vi "FGV Slit.vi"(8 "error in (no error)":errorcluster, 10 "FGV Slit Data In":T1 {"Système ID" min=1 max=10 step=1; "Portnumber" items=["COM1", "COM2", "COM3", "COM4", "COM5", "COM6", "COM7", "COM8", "COM9", "COM10", "COM11", "COM12", "COM13", "COM14", "COM15", "COM16", "COM17", "COM18", "COM19", "COM20", "COM21", "COM22", "COM23", "COM24", "COM25", "COM26", "COM27", "COM28", "COM29", "COM30"]}, 11 "Action":T2) -> (0 "error out":errorcluster, 3 "FGV Slit Data Out":T1={"Portnumber"=0, "Position"=0.0, "Status"="", "Système ID"=1, "Connected axes"=[], "Velocity"=0.0, "Stage names"=[], "Device ID out"=0} {"Système ID" min=1 max=10 step=1; "Portnumber" items=["COM1", "COM2", "COM3", "COM4", "COM5", "COM6", "COM7", "COM8", "COM9", "COM10", "COM11", "COM12", "COM13", "COM14", "COM15", "COM16", "COM17", "COM18", "COM19", "COM20", "COM21", "COM22", "COM23", "COM24", "COM25", "COM26", "COM27", "COM28", "COM29", "COM30"]})   [LabVIEW 2017]
uses:
  Action Slit.ctl
  FGV Slit Data.ctl
  <userlib>/GCSLabView/Low Level/Communication.llb/Available interfaces.ctl
  <userlib>/GCSLabView/Low Level/Communication.llb/Available DLLs.ctl
  <userlib>/GCSLabView/Low Level/Communication.llb/Available DLL interfaces.ctl
  <userlib>/GCSLabView/Low Level/General command.llb/Controller names.ctl
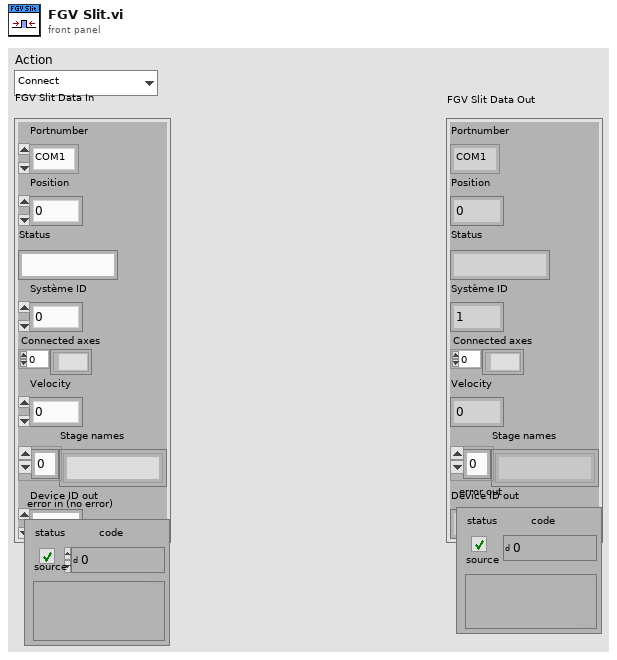
[diagram p1: front panel]
types:
  T1 = typedef "FGV Slit Data.ctl" = cluster{"Portnumber":i32, "Position":dbl, "Status":string, "Système ID":i32, "Connected axes":string[], "Velocity":dbl, "Stage names":string[], "Device ID out":i32}
  T2 = typedef "Action Slit.ctl" = enum16{"Connect", "Initialize", "Set Velocity", "Get Velocity", "Move Rel", "Move Abs", "Position", "Status", "Abort", "Disconnect"}
  T3 = typedef "Available interfaces.ctl" = u16
  T4 = cluster{"RS232 Portnumber":i32, "Timeout":i32, "RS232 Baud rate":u32, "Interface":T3, "GPIB Bus":i32, "GPIB Address":i32, "GPIB Mode":i32}
  T5 = cluster{"input XON/XOFF":bool, "input HW Handshake":bool, "input alt HW HShk":bool, "output XON/XOFF":bool, "output HW Handshake":bool, "output alt HW HShk":bool, "XOFF byte ":u8, "XON byte":u8, "parity error byte":u16}
  T6 = cluster{"data bits":u16, "stop bits":enum16{"1 bit", "1.5 bits", "2 bits"}, "parity":enum16{"no parity", "odd parity", "even parity", "mark parity", "space parity"}}
  T7 = typedef "Controller names.ctl" = enum16{"None", "Analog", "C-702", "C-843", "C-843.PM", "C-844", "C-848", "C-865", "C-866", "C-867", "C-880", "E-516", "E-517", "E-709", "E-710", "E-712", "E-725", "E-753", "E-755", "E-761", "E-816", "E-861", "F-206", "M-840", "M-850", "M-8X0", "Mercury", "Mercury_GCS"}
  T8 = typedef "Available DLLs.ctl" = u16
  T9 = typedef "Available DLL interfaces.ctl" = u16
  T10 = cluster{"DLL for Device":T8, "DLL Interface":T9, "Parameter":string}
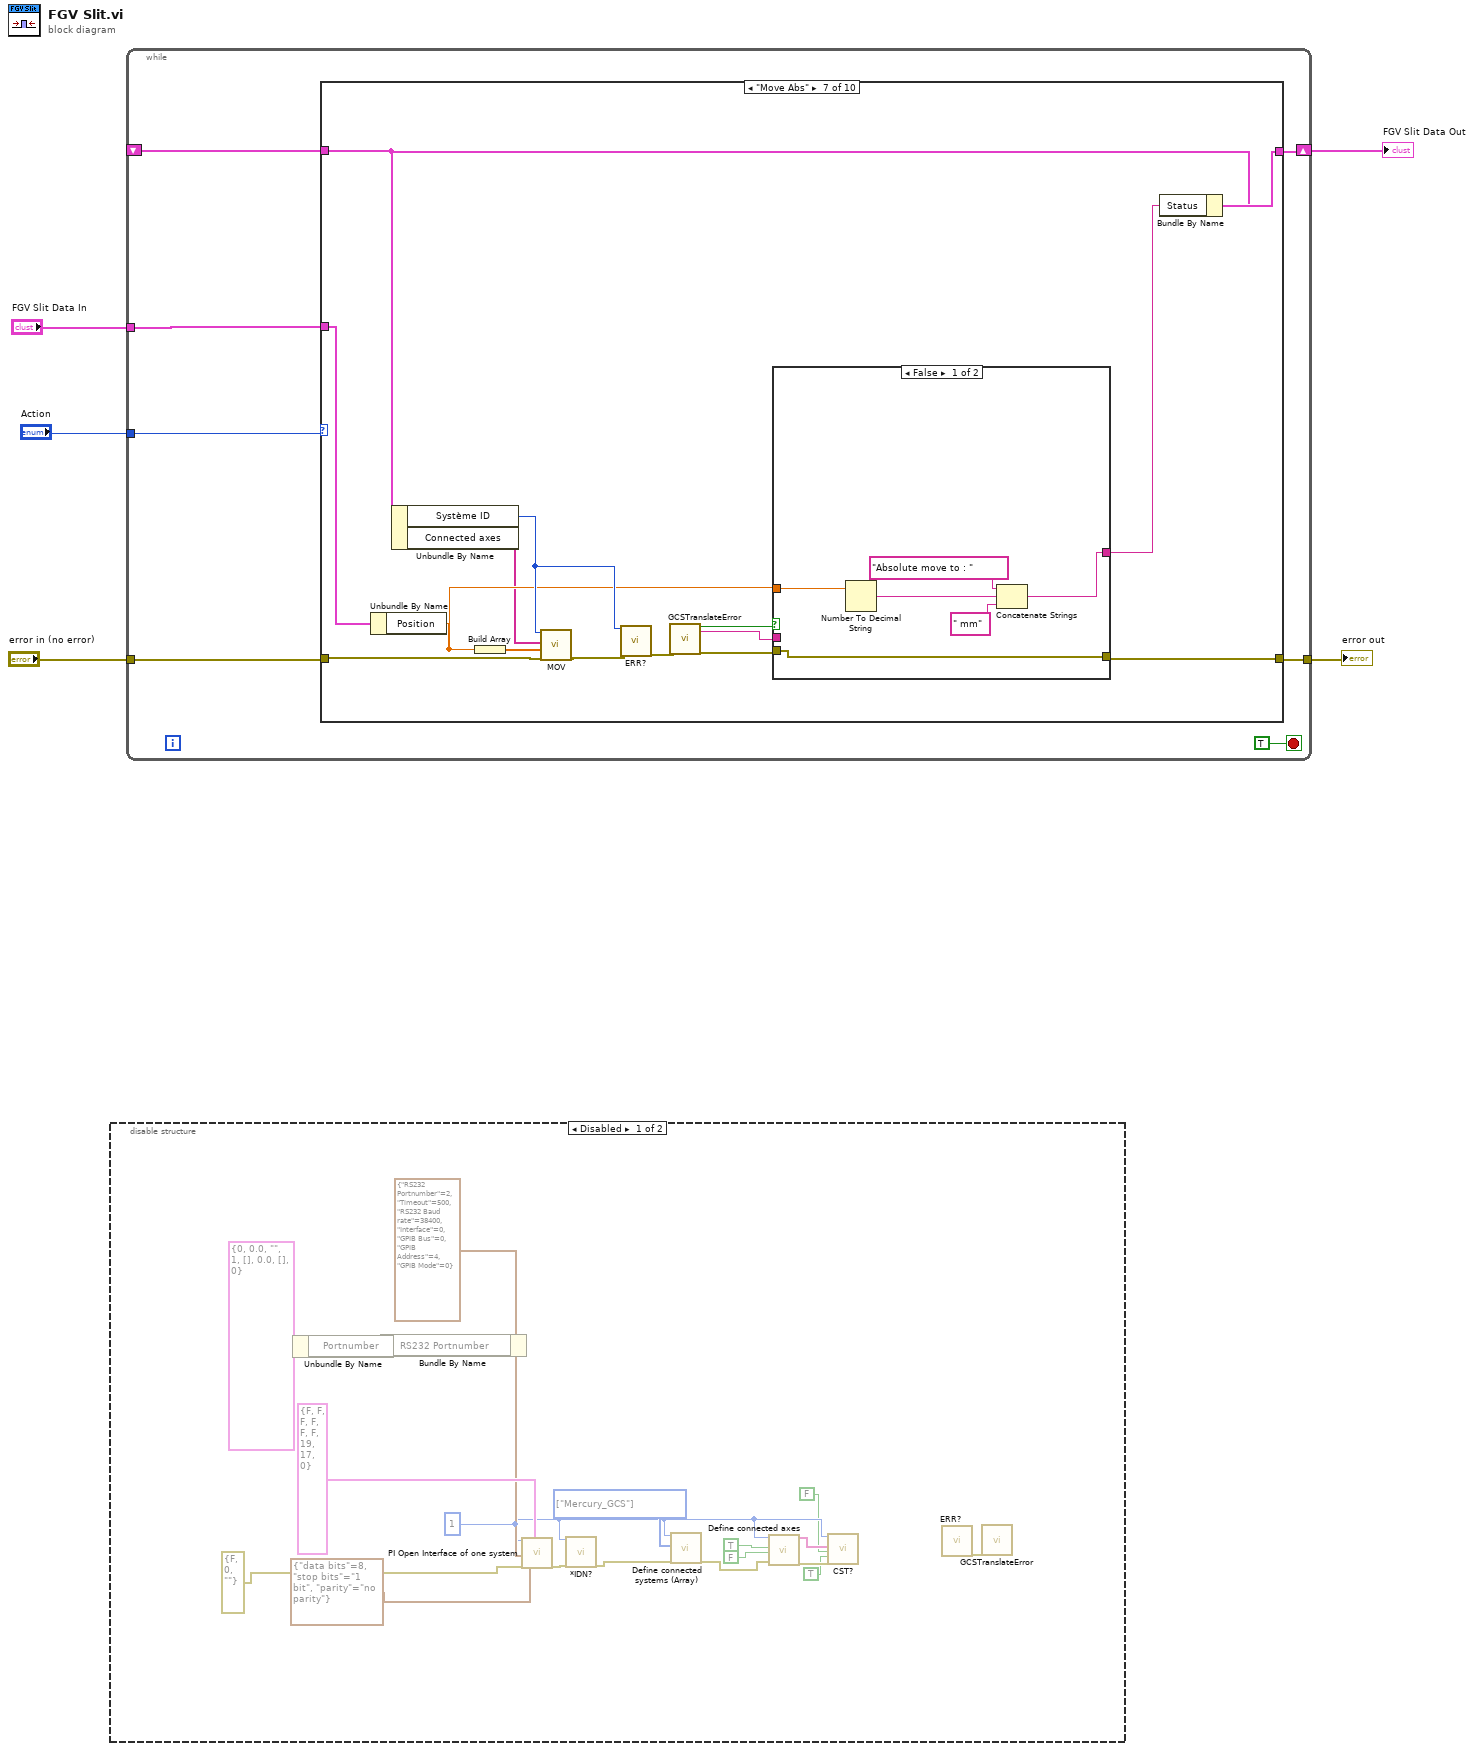
[diagram p0: block diagram]
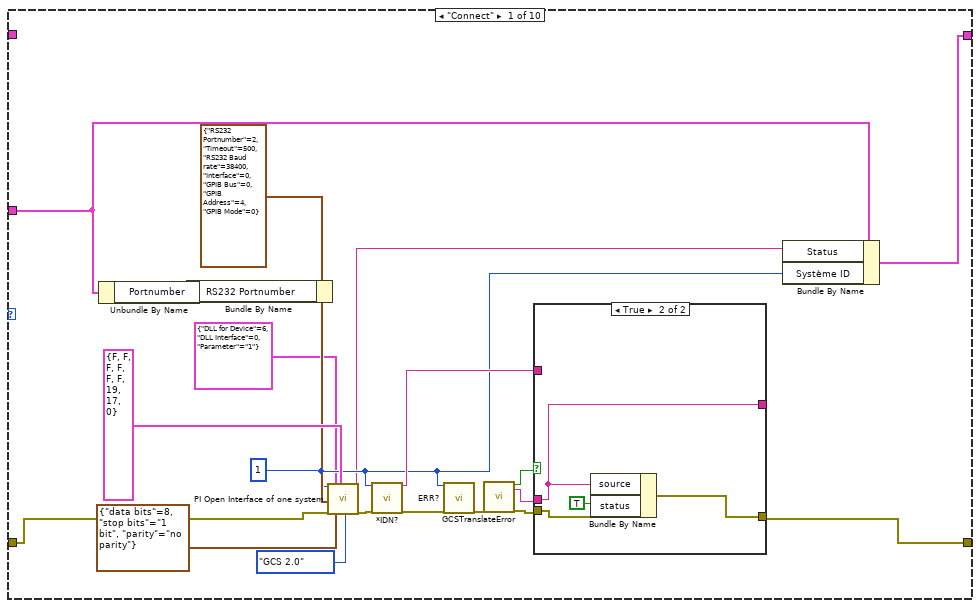
[diagram p3: hidden frame]
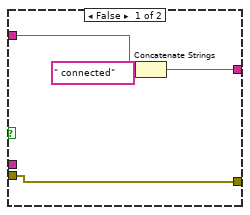
[diagram p4: hidden frame]
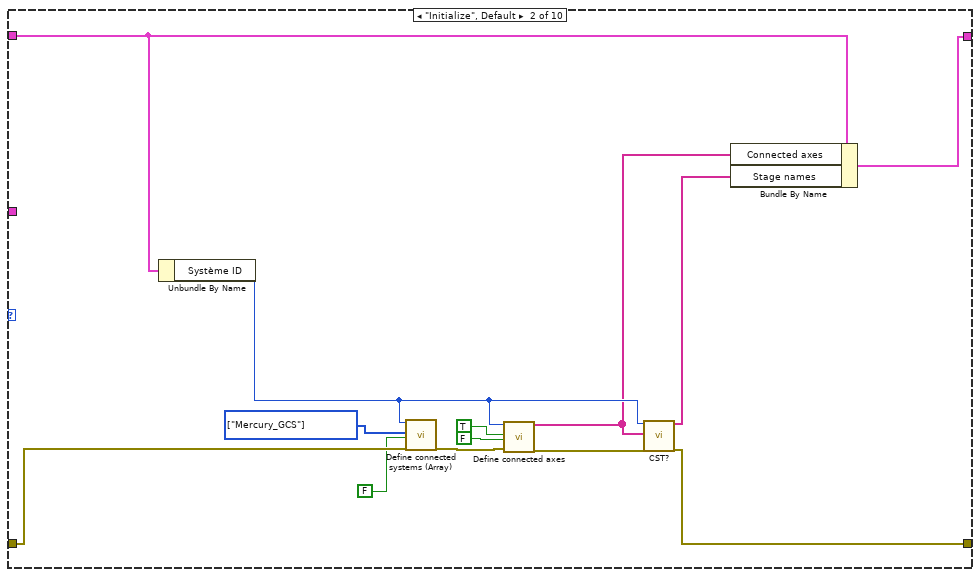
[diagram p5: hidden frame]
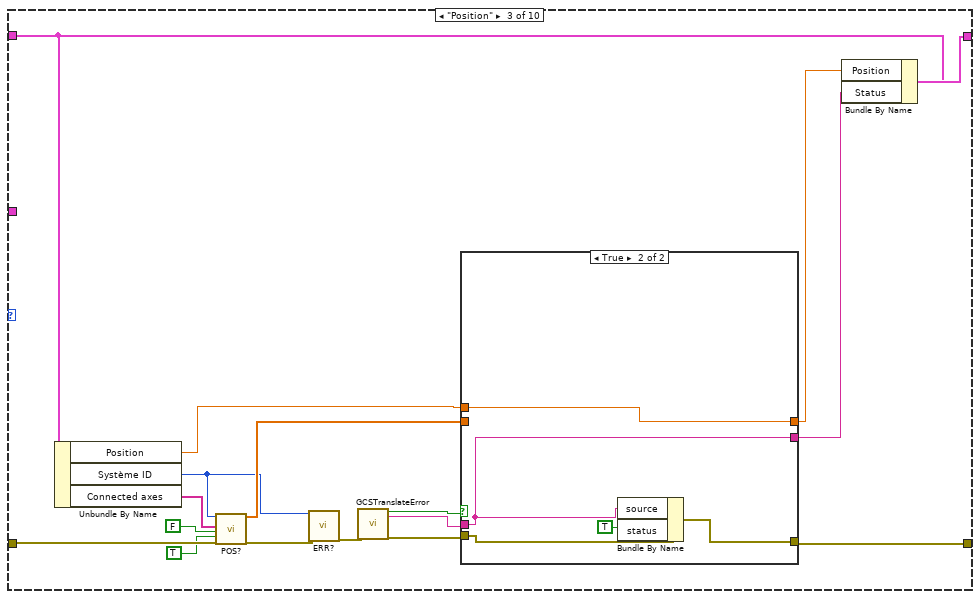
[diagram p6: hidden frame]
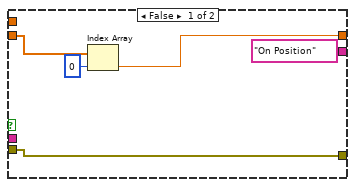
[diagram p7: hidden frame]
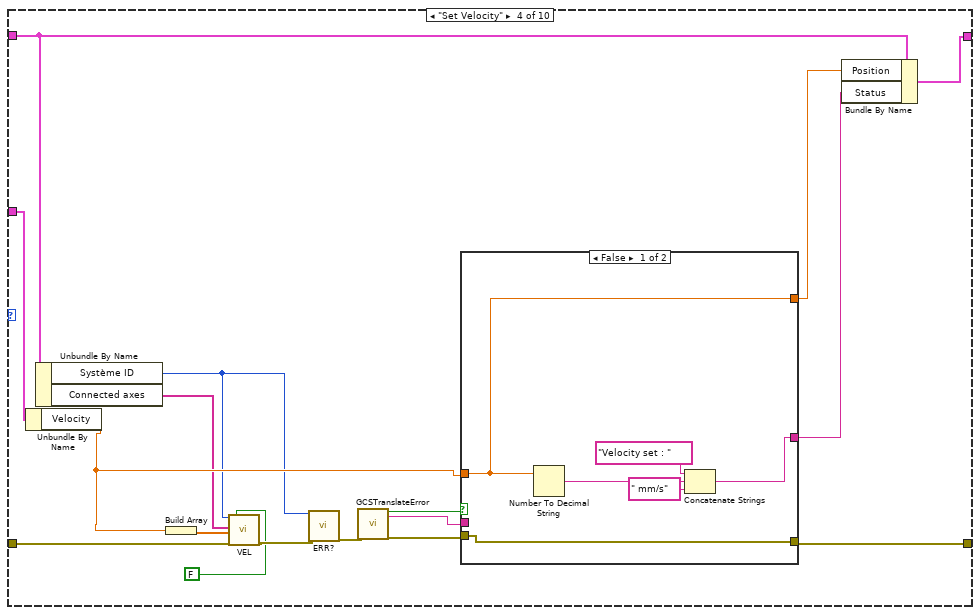
[diagram p8: hidden frame]
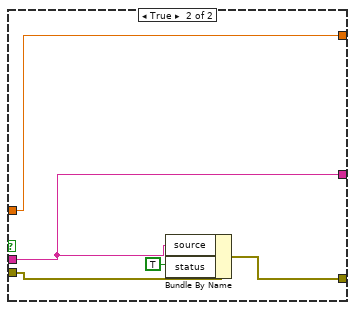
[diagram p9: hidden frame]
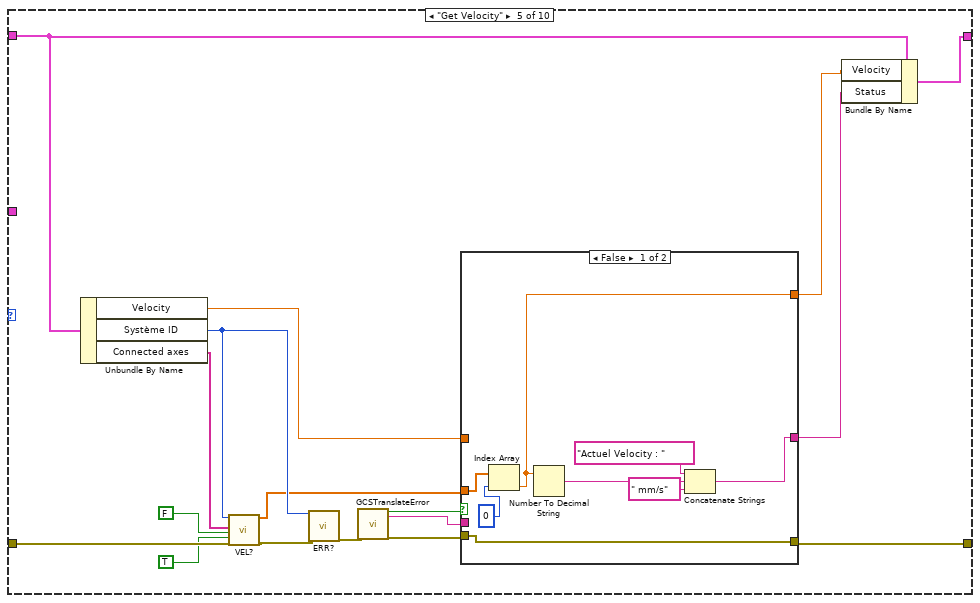
[diagram p10: hidden frame]
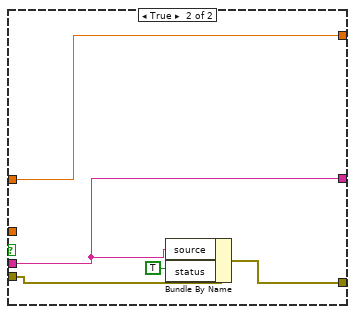
[diagram p11: hidden frame]
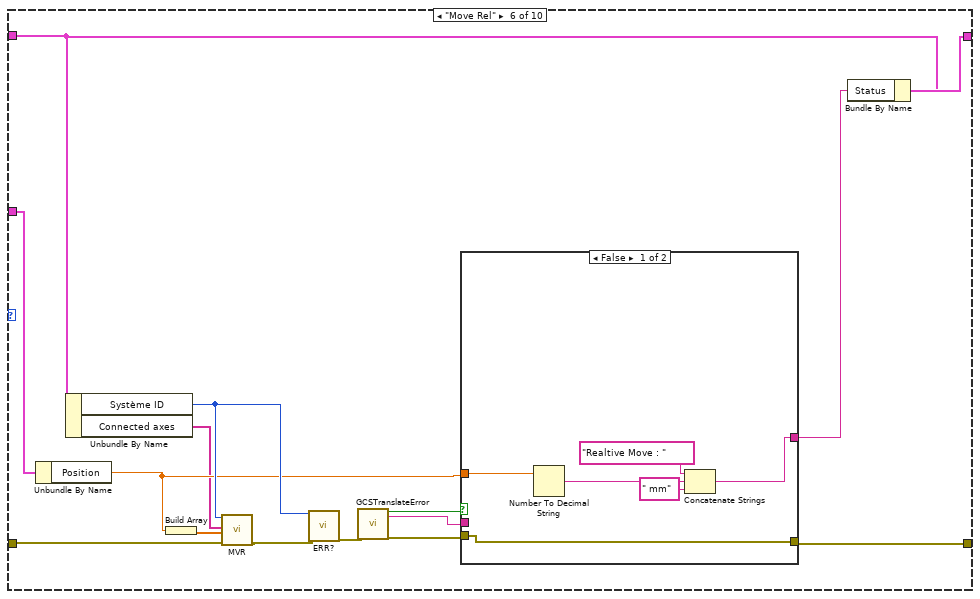
[diagram p12: hidden frame]
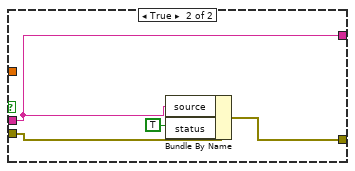
[diagram p13: hidden frame]
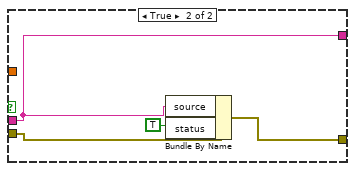
[diagram p14: hidden frame]
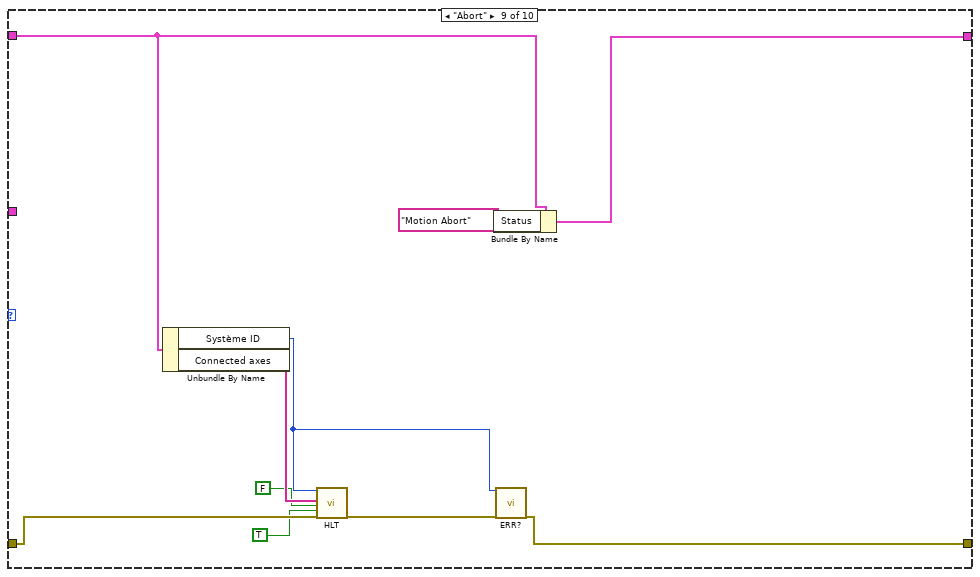
[diagram p16: hidden frame]
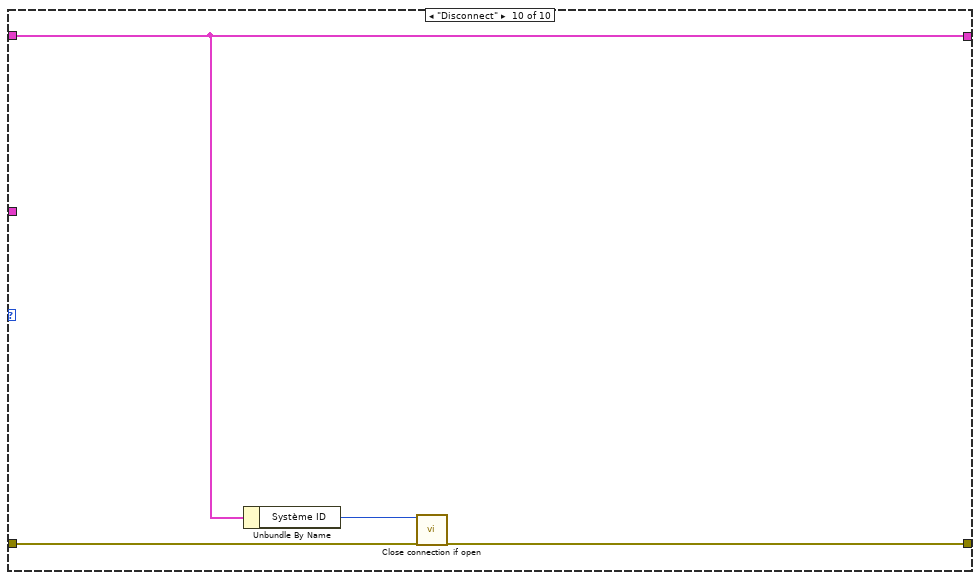
[diagram p17: hidden frame]
diagram:
  n1 = disable-structure shown="Disabled" {
    frame Disabled {
      w18 = T7[] [enum."Mercury_GCS"] items=["None", "Analog", "C-702", "C-843", "C-843.PM", "C-844", "C-848", "C-865", "C-866", "C-867", "C-880", "E-516", "E-517", "E-709", "E-710", "E-712", "E-725", "E-753", "E-755", "E-761", "E-816", "E-861", "F-206", "M-840", "M-850", "M-8X0", "Mercury", "Mercury_GCS"] ("Controller names")
      w10 = 1 ("System number")
      n2 = Unbundle By Name(T1 {"Portnumber"=0, "Position"=0.0, "Status"="", "Système ID"=1, "Connected axes"=[], "Velocity"=0.0, "Stage names"=[], "Device ID out"=0} ("input cluster")) -> ("Portnumber"=w20:i32)
      n3 = Bundle By Name(cluster=T4 {"RS232 Portnumber"=2, "Timeout"=500, "RS232 Baud rate"=38400, "Interface"=0, "GPIB Bus"=0, "GPIB Address"=4, "GPIB Mode"=0} ("Interface configuration"), "RS232 Portnumber"=w20) -> (w19:T4)
      n4 = call <userlib>:"PI Open Interface of one system.vi"("System number"=w10, "Interface configuration"=w19, "error in"=errorcluster {"status"=FALSE, "code"=0, "source"=""}, "Bit settings and parity"=T6 {"data bits"=8, "stop bits"=enum."1 bit", "parity"=enum."no parity"}, "Flow control"=T5 {"input XON/XOFF"=FALSE, "input HW Handshake"=FALSE, "input alt HW HShk"=FALSE, "output XON/XOFF"=FALSE, "output HW Handshake"=FALSE, "output alt HW HShk"=FALSE, "XOFF byte "=19, "XON byte"=17, "parity error byte"=0}) -> ("error out"=w22:errorcluster)  [unwired: 13 in, 1 out]
      n5 = call <userlib>:"*IDN?.vi"("System no."=w10, "error in"=w22) -> ("error out"=w14:errorcluster)  [unwired: 16 in, 1 out]
      n6 = call <userlib>:"Define connected systems (Array).vi"("System no."=w10, "Controller names"=w18, "error in"=w14) -> ("error out"=w11:errorcluster)  [unwired: 16 in]
      n7 = call <userlib>:"Define connected axes.vi"("System no."=w10, "Read from\ncontroller?"=TRUE ("Read from\ncontroller?"), "Invert\norder?"=FALSE ("Invert\norder?"), "error in"=w11) -> ("Conn. Axes out"=w9:string[], "error out"=w8:errorcluster)  [unwired: 14 in]
      n8 = call <userlib>:"CST?.vi"("System no."=w10, "Axes to query"=w9, "All Axes?"=FALSE, "Axis Identifier?"=TRUE, "error in"=w8) -> ()  [unwired: 13 in, 2 out]
      n9 = call <userlib>:"ERR?.vi"() -> ("error out"=w24:errorcluster)  [unwired: 18 in, 1 out]
      n10 = call <userlib>:"GCSTranslateError.vi"("error in"=w24) -> ()  [unwired: 16 in, 3 out]
    }
    frame Enabled {
    }
  }
  n11 = while {
    tunnel: "Action" -> [w30]
    tunnel: "FGV Slit Data In" -> [w29]
    shift-right: [w28] -> w3
    shift-left: _ -> [w25]
    tunnel: "error in (no error)" -> [w27]
    tunnel: [w26] -> w1
    stop <- TRUE stop-if-true
    n12 = case shown="\"Move Abs\"" w30 {
      tunnel: w29 -> [w48 _ _ w105 _ w160 w185 _ _ _]
      tunnel: [w50 w62 w85 w112 w140 w168 w193 w209 w213 w222] -> w28
      tunnel: w25 -> [_ w64 w81 w102 w130 w161 w186 w209 w215 w222]
      tunnel: w27 -> [w49 w67 w83 w108 w136 w165 w189 w208 w219 w223]
      tunnel: [w51 w66 w84 w111 w139 w167 w192 w208 w217 w220] -> w26
      frame "Connect" {
        w36 = 1 ("System number")
        n13 = Unbundle By Name(w48) -> ("Portnumber"=w38:i32)
        n14 = Bundle By Name(cluster=T4 {"RS232 Portnumber"=2, "Timeout"=500, "RS232 Baud rate"=38400, "Interface"=0, "GPIB Bus"=0, "GPIB Address"=4, "GPIB Mode"=0} ("Interface configuration"), "RS232 Portnumber"=w38) -> (w37:T4)
        n15 = call <userlib>:"PI Open Interface of one system.vi"("System number"=w36, "Interface configuration"=w37, "error in"=w49, "DLL Interface\nConfiguration"=T10 {"DLL for Device"=6, "DLL Interface"=0, "Parameter"="1"} ("DLL Interface\nConfiguration"), "Bit settings and parity"=T6 {"data bits"=8, "stop bits"=enum."1 bit", "parity"=enum."no parity"}, "Flow control"=T5 {"input XON/XOFF"=FALSE, "input HW Handshake"=FALSE, "input alt HW HShk"=FALSE, "output XON/XOFF"=FALSE, "output HW Handshake"=FALSE, "output alt HW HShk"=FALSE, "XOFF byte "=19, "XON byte"=17, "parity error byte"=0}, "Syntax"=enum16{"GCS 1.0", "GCS 2.0"}."GCS 2.0") -> ("String read"=w33:string, "error out"=w41:errorcluster)  [unwired: 11 in]
        n16 = call <userlib>:"*IDN?.vi"("System no."=w36, "error in"=w41) -> ("Identification"=w40:string, "error out"=w35:errorcluster)  [unwired: 16 in]
        n17 = call <userlib>:"ERR?.vi"("System no."=w36, "error in"=w35) -> ("error out"=w47:errorcluster)  [unwired: 16 in, 1 out]
        n18 = call <userlib>:"GCSTranslateError.vi"("error in"=w47) -> ("GCS Error?"=w46:bool, "Error Description"=w45:string, "error out"=w44:errorcluster)  [unwired: 16 in]
        n19 = case shown="True" w46 {
          tunnel: w40 -> [w55 _]
          tunnel: [w52 w58] -> w51
          tunnel: [w53 w57] -> _
          tunnel: w45 -> [_ w57]
          tunnel: w44 -> [w52 w59]
          frame False {
            n20 = Concatenate Strings(w55, " connected" ("string")) -> (w53:string)
          }
          frame True {
            n21 = Bundle By Name(cluster=w59, "source"=w57, "status"=TRUE) -> (w58:errorcluster)
          }
        }
        n22 = Bundle By Name(cluster=w48, "Status"=w33, "Système ID"=w36) -> (w50:T1)
      }
      frame "Initialize", Default {
        w72 = T7[] [enum."Mercury_GCS"] items=["None", "Analog", "C-702", "C-843", "C-843.PM", "C-844", "C-848", "C-865", "C-866", "C-867", "C-880", "E-516", "E-517", "E-709", "E-710", "E-712", "E-725", "E-753", "E-755", "E-761", "E-816", "E-861", "F-206", "M-840", "M-850", "M-8X0", "Mercury", "Mercury_GCS"] ("Controller names")
        n23 = Unbundle By Name(w64) -> ("Système ID"=w65:i32)
        n24 = call <userlib>:"Define connected systems (Array).vi"("System no."=w65, "Controller names"=w72, "Change only one system?"=FALSE, "error in"=w67) -> ("error out"=w69:errorcluster)  [unwired: 15 in]
        n25 = call <userlib>:"Define connected axes.vi"("System no."=w65, "Read from\ncontroller?"=TRUE ("Read from\ncontroller?"), "Invert\norder?"=FALSE ("Invert\norder?"), "error in"=w69) -> ("Conn. Axes out"=w60:string[], "error out"=w68:errorcluster)  [unwired: 14 in]
        n26 = call <userlib>:"CST?.vi"("System no."=w65, "Axes to query"=w60, "error in"=w68) -> ("Stage names"=w63:string[], "error out"=w66:errorcluster)  [unwired: 15 in]
        n27 = Bundle By Name(cluster=w64, "Connected axes"=w60, "Stage names"=w63) -> (w62:T1)
      }
      frame "Position" {
        n28 = Unbundle By Name(w81) -> ("Position"=w79:dbl, "Système ID"=w75:i32, "Connected axes"=w76:string[])
        n29 = call <userlib>:"POS?.vi"("System no."=w75, "Axes to query"=w76, "All axes?"=FALSE, "Axis identifier?"=TRUE, "error in"=w83) -> ("Position"=w80:dbl[], "error out"=w82:errorcluster)  [unwired: 13 in]
        n30 = call <userlib>:"ERR?.vi"("System no."=w75, "error in"=w82) -> ("error out"=w89:errorcluster)  [unwired: 16 in, 1 out]
        n31 = call <userlib>:"GCSTranslateError.vi"("error in"=w89) -> ("GCS Error?"=w88:bool, "Error Description"=w87:string, "error out"=w86:errorcluster)  [unwired: 16 in]
        n32 = case shown="True" w88 {
          tunnel: [w94 w98] -> w84
          tunnel: ["On Position" ("Error Description") w97] -> w78
          tunnel: w87 -> [_ w97]
          tunnel: w86 -> [w94 w99]
          tunnel: w80 -> [w92 _]
          tunnel: [w90 w95] -> w77
          tunnel: w79 -> [_ w95]
          frame False {
            n33 = Index Array(array=w92, index=0) -> (element=w90:dbl)
          }
          frame True {
            n34 = Bundle By Name(cluster=w99, "source"=w97, "status"=TRUE) -> (w98:errorcluster)
          }
        }
        n35 = Bundle By Name(cluster=w81, "Position"=w77, "Status"=w78) -> (w85:T1)
      }
      frame "Set Velocity" {
        n36 = Unbundle By Name(w105) -> ("Velocity"=w104:dbl)
        n37 = Unbundle By Name(w102) -> ("Système ID"=w103:i32, "Connected axes"=w100:string[])
        n38 = Build Array(w104) -> (w109:dbl[])
        n39 = call <userlib>:"VEL.vi"("System no."=w103, "Axes to set"=w100, "Velocity values"=w109, "error in"=w108, "Without axis ID?"=FALSE) -> ("error out"=w107:errorcluster)  [unwired: 13 in, 1 out]
        n40 = call <userlib>:"ERR?.vi"("System no."=w103, "error in"=w107) -> ("error out"=w116:errorcluster)  [unwired: 16 in, 1 out]
        n41 = call <userlib>:"GCSTranslateError.vi"("error in"=w116) -> ("GCS Error?"=w115:bool, "Error Description"=w114:string, "error out"=w113:errorcluster)  [unwired: 16 in]
        n42 = case shown="False" w115 {
          tunnel: [w122 w126] -> w111
          tunnel: [w119 w125] -> w110
          tunnel: w114 -> [_ w125]
          tunnel: w113 -> [w122 w127]
          tunnel: w104 -> [w117 w123]
          tunnel: [w117 w123] -> w106
          frame False {
            n43 = Number To Decimal String(number=w117) -> (decimal integer string=w121:string)  [unwired: 1 in]
            n44 = Concatenate Strings("Velocity set : " ("Error Description"), w121, " mm/s" ("string")) -> (w119:string)
          }
          frame True {
            n45 = Bundle By Name(cluster=w127, "source"=w125, "status"=TRUE) -> (w126:errorcluster)
          }
        }
        n46 = Bundle By Name(cluster=w102, "Position"=w106, "Status"=w110) -> (w112:T1)
      }
      frame "Get Velocity" {
        n47 = Unbundle By Name(w130) -> ("Velocity"=w131:dbl, "Système ID"=w137:i32, "Connected axes"=w133:string[])
        n48 = call <userlib>:"VEL?.vi"("System no."=w137, "Axes to query"=w133, "All axes?"=FALSE, "Axis identifier?"=TRUE, "error in"=w136) -> ("Velocity"=w134:dbl[], "error out"=w135:errorcluster)  [unwired: 13 in]
        n49 = call <userlib>:"ERR?.vi"("System no."=w137, "error in"=w135) -> ("error out"=w144:errorcluster)  [unwired: 16 in, 1 out]
        n50 = call <userlib>:"GCSTranslateError.vi"("error in"=w144) -> ("GCS Error?"=w143:bool, "Error Description"=w142:string, "error out"=w141:errorcluster)  [unwired: 16 in]
        n51 = case shown="False" w143 {
          tunnel: [w152 w156] -> w139
          tunnel: [w149 w155] -> w138
          tunnel: w142 -> [_ w155]
          tunnel: w141 -> [w152 w157]
          tunnel: w134 -> [w147 _]
          tunnel: [w145 w153] -> w132
          tunnel: w131 -> [_ w153]
          frame False {
            n52 = Index Array(array=w147, index=i16 0 ("width (-)")) -> (element=w145:dbl)
            n53 = Number To Decimal String(number=w145) -> (decimal integer string=w151:string)  [unwired: 1 in]
            n54 = Concatenate Strings("Actuel Velocity : " ("Error Description"), w151, " mm/s" ("string")) -> (w149:string)
          }
          frame True {
            n55 = Bundle By Name(cluster=w157, "source"=w155, "status"=TRUE) -> (w156:errorcluster)
          }
        }
        n56 = Bundle By Name(cluster=w130, "Velocity"=w132, "Status"=w138) -> (w140:T1)
      }
      frame "Move Rel" {
        n57 = Unbundle By Name(w160) -> ("Position"=w159:dbl)
        n58 = Unbundle By Name(w161) -> ("Système ID"=w162:i32, "Connected axes"=w158:string[])
        n59 = Build Array(w159) -> (w163:dbl[])
        n60 = call <userlib>:"MVR.vi"("System no."=w162, "Axes to move"=w158, "Position values"=w163, "error in"=w165) -> ("error out"=w164:errorcluster)  [unwired: 15 in]
        n61 = call <userlib>:"ERR?.vi"("System no."=w162, "error in"=w164) -> ("error out"=w172:errorcluster)  [unwired: 16 in, 1 out]
        n62 = call <userlib>:"GCSTranslateError.vi"("error in"=w172) -> ("GCS Error?"=w171:bool, "Error Description"=w170:string, "error out"=w169:errorcluster)  [unwired: 16 in]
        n63 = case shown="False" w171 {
          tunnel: [w178 w181] -> w167
          tunnel: [w174 w180] -> w166
          tunnel: w170 -> [_ w180]
          tunnel: w169 -> [w178 w182]
          tunnel: w159 -> [w177 _]
          frame False {
            n64 = Number To Decimal String(number=w177) -> (decimal integer string=w176:string)  [unwired: 1 in]
            n65 = Concatenate Strings("Realtive Move : " ("Error Description"), w176, " mm" ("string")) -> (w174:string)
          }
          frame True {
            n66 = Bundle By Name(cluster=w182, "source"=w180, "status"=TRUE) -> (w181:errorcluster)
          }
        }
        n67 = Bundle By Name(cluster=w161, "Status"=w166) -> (w168:T1)
      }
      frame "Move Abs" {
        n68 = Unbundle By Name(w185) -> ("Position"=w184:dbl)
        n69 = Unbundle By Name(w186) -> ("Système ID"=w187:i32, "Connected axes"=w183:string[])
        n70 = Build Array(w184) -> (w188:dbl[])
        n71 = call <userlib>:"MOV.vi"("System no."=w187, "Axes to move"=w183, "Position values"=w188, "error in"=w189) -> ("error out"=w190:errorcluster)  [unwired: 15 in]
        n72 = call <userlib>:"ERR?.vi"("System no."=w187, "error in"=w190) -> ("error out"=w197:errorcluster)  [unwired: 16 in, 1 out]
        n73 = call <userlib>:"GCSTranslateError.vi"("error in"=w197) -> ("GCS Error?"=w196:bool, "Error Description"=w195:string, "error out"=w194:errorcluster)  [unwired: 16 in]
        n74 = case shown="False" w196 {
          tunnel: [w203 w206] -> w192
          tunnel: [w199 w205] -> w191
          tunnel: w195 -> [_ w205]
          tunnel: w194 -> [w203 w207]
          tunnel: w184 -> [w202 _]
          frame False {
            n75 = Number To Decimal String(number=w202) -> (decimal integer string=w201:string)  [unwired: 1 in]
            n76 = Concatenate Strings("Absolute move to : " ("Error Description"), w201, " mm" ("string")) -> (w199:string)
          }
          frame True {
            n77 = Bundle By Name(cluster=w207, "source"=w205, "status"=TRUE) -> (w206:errorcluster)
          }
        }
        n78 = Bundle By Name(cluster=w186, "Status"=w191) -> (w193:T1)
      }
      frame "Status" {
      }
      frame "Abort" {
        n79 = Unbundle By Name(w215) -> ("Système ID"=w216:i32, "Connected axes"=w212:string[])
        n80 = call <userlib>:"HLT.vi"("System no."=w216, "Affected axes"=w212, "All axes?"=FALSE, "Axis identifier?"=TRUE, "error in"=w219) -> ("error out"=w218:errorcluster)  [unwired: 14 in]
        n81 = Bundle By Name(cluster=w215, "Status"="Motion Abort") -> (w213:T1)
        n82 = call <userlib>:"ERR?.vi"("System no."=w216, "error in"=w218) -> ("error out"=w217:errorcluster)  [unwired: 16 in, 1 out]
      }
      frame "Disconnect" {
        n83 = Unbundle By Name(w222) -> ("Système ID"=w221:i32)
        n84 = call <userlib>:"Close connection if open.vi"("System no."=w221, "error in"=w223) -> ("error out"=w220:errorcluster)  [unwired: 16 in, 1 out]
      }
    }
  }
  "FGV Slit Data Out" <- w3
  "error out" <- w1
